vi "3_Axis_magmeter_MAIN.vi"() -> ()   [LabVIEW 2013]
doc: "Программа для обработки и визуализации трех компонент магнитного поля прибора, разработаного инженерами НЭОиКН ЛФВЭ ОИЯИ 2014"
uses:
  Magmeter.ctl
  <vilib>/Instr/_visa.llb/VISA Configure Serial Port (Instr).vi
panel:
  out "Dx Sum":u64
  in  "Порт":refnum<visa-resource-name>="COM4"
  out "Соединение":bool
  out "Err msg":string=" INSTRUCTIONS:\r\rNormal Use:  When using subVIs that incorporate the error in/error out (or error I/O) structure, place this handler where you want to inform the user of an error, typically at the end of the I/O data path, as the last action of the program.  If the error in error? is ERROR, the handler creates a message describing the error and its source.  If the type of dialog = 1 (default), the message is displayed to the user, who can only acknowedge it.  If the type = 2, the user can acknowledge the message or abort execution; aborting a program with active I/O is not recommended.  If the type = 0, no message is displayed; this is used to process the error programmatically, and the error out cluster elements are wired to individual terminals for that reason.  \r\rOther Use:\n\r\nlocal testing.  To test the error code of a subVI or function that does not have the error I/O structure, you can wire its error code and a source string to the local error code and error source inputs.  If error in error? indicates no error and error code is not equal to 0, the local code and source are substituted for the error in values, and error? is set TRUE (ERROR)."
  in  "Бод.":u32=9600
  out "i":i32
  in  "number of data sample":u64
  in  "Маркеры":bool
  out "Table num index":u32
  in  "Удалить измерение":bool
  in  "RXd number":u64
  in  "Dz, мм":u64=5 min=1
  in  "зафиксировать измерение":bool
  in  "Измерений \nна графике":u16=100
  in  "Очистить историю":bool
  in  "H макс":dbl=8.0 format="%#.1f"
  in  "H мин":dbl=-8.0 format="%#.1f"
  in  "Уст. ноль":bool
  in  "Сохранен!":bool
  in  "Plot.Visible Z":bool
  out "By":dbl format="%.3f"
  out "Bz":dbl format="%.3f"
  in  "Plot.Visible X":bool
  out "Bx":dbl format="%.3f"
  in  "Plot.Visible Y":bool
  in  "Графики толще":bool=TRUE
  in  "Scale Max, Ga":string(combo)="8,1"
  in  "Стоп":bool
  out "Магнитные измерения":T1(graph)
  in  "Measurment Fl":bool
  out "Сохраненные измерения":string[][](table)
  out "Путь к файлу":path
  # "Гаусс"
  # "Результаты\nизмерений"
  # "ГС"
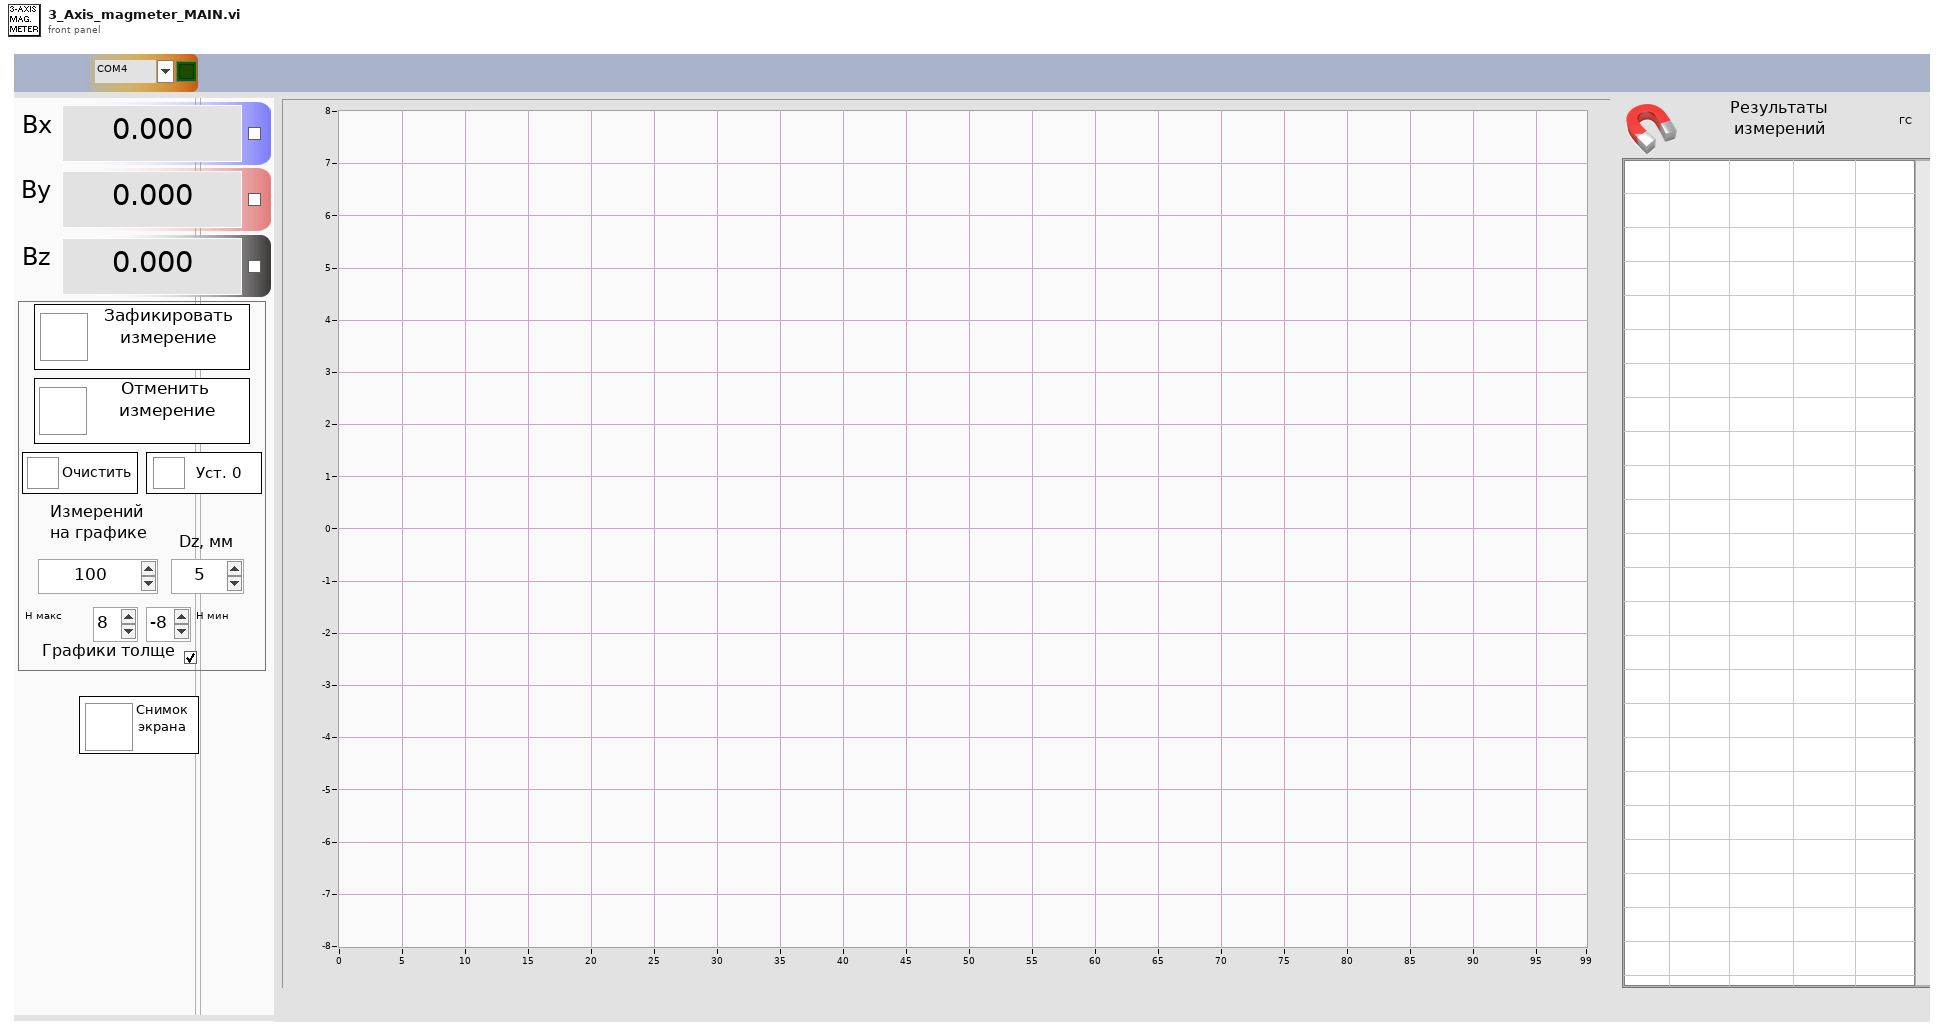
[diagram p1: front panel]
types:
  T1 = cluster{"X":dbl, "Y":dbl, "Z":dbl, "Active Plot":dbl}[]
  T2 = typedef "Magmeter.ctl" = enum16{"Initialize", "Read port", "Write port", "Stop"}
  T3 = cluster{"Value":dbl, "Value":dbl, "Value":dbl, "Active Plot":dbl}
  T4 = cluster{"Value":dbl, "Value":dbl, "Value":dbl, "X":dbl}
  T5 = cluster{"Value":dbl, "Value":dbl, "Value":dbl, "X":dbl}[]
  T6 = typedef "imagedata.ctl" = cluster{"image type":i32, "image depth":i32, "image":u8[], "mask":u8[], "colors":u32[], "Rectangle":cluster{"left":i16, "top":i16, "right":i16, "bottom":i16}}
  T7 = cluster{"read buffer":string, "serial out":refnum<visa-resource-name>, "error out":errorcluster, "occurrence":refnum<k4>}
  T8 = cluster{"Scale Max out ":string, "out string":string, "Visa name out":refnum<visa-resource-name>, "error out":errorcluster, "occurrence":refnum<k4>}
  T9 = cluster{"Visa name out":refnum<visa-resource-name>, "error out":errorcluster, "status":bool, "occurrence":refnum<k4>}
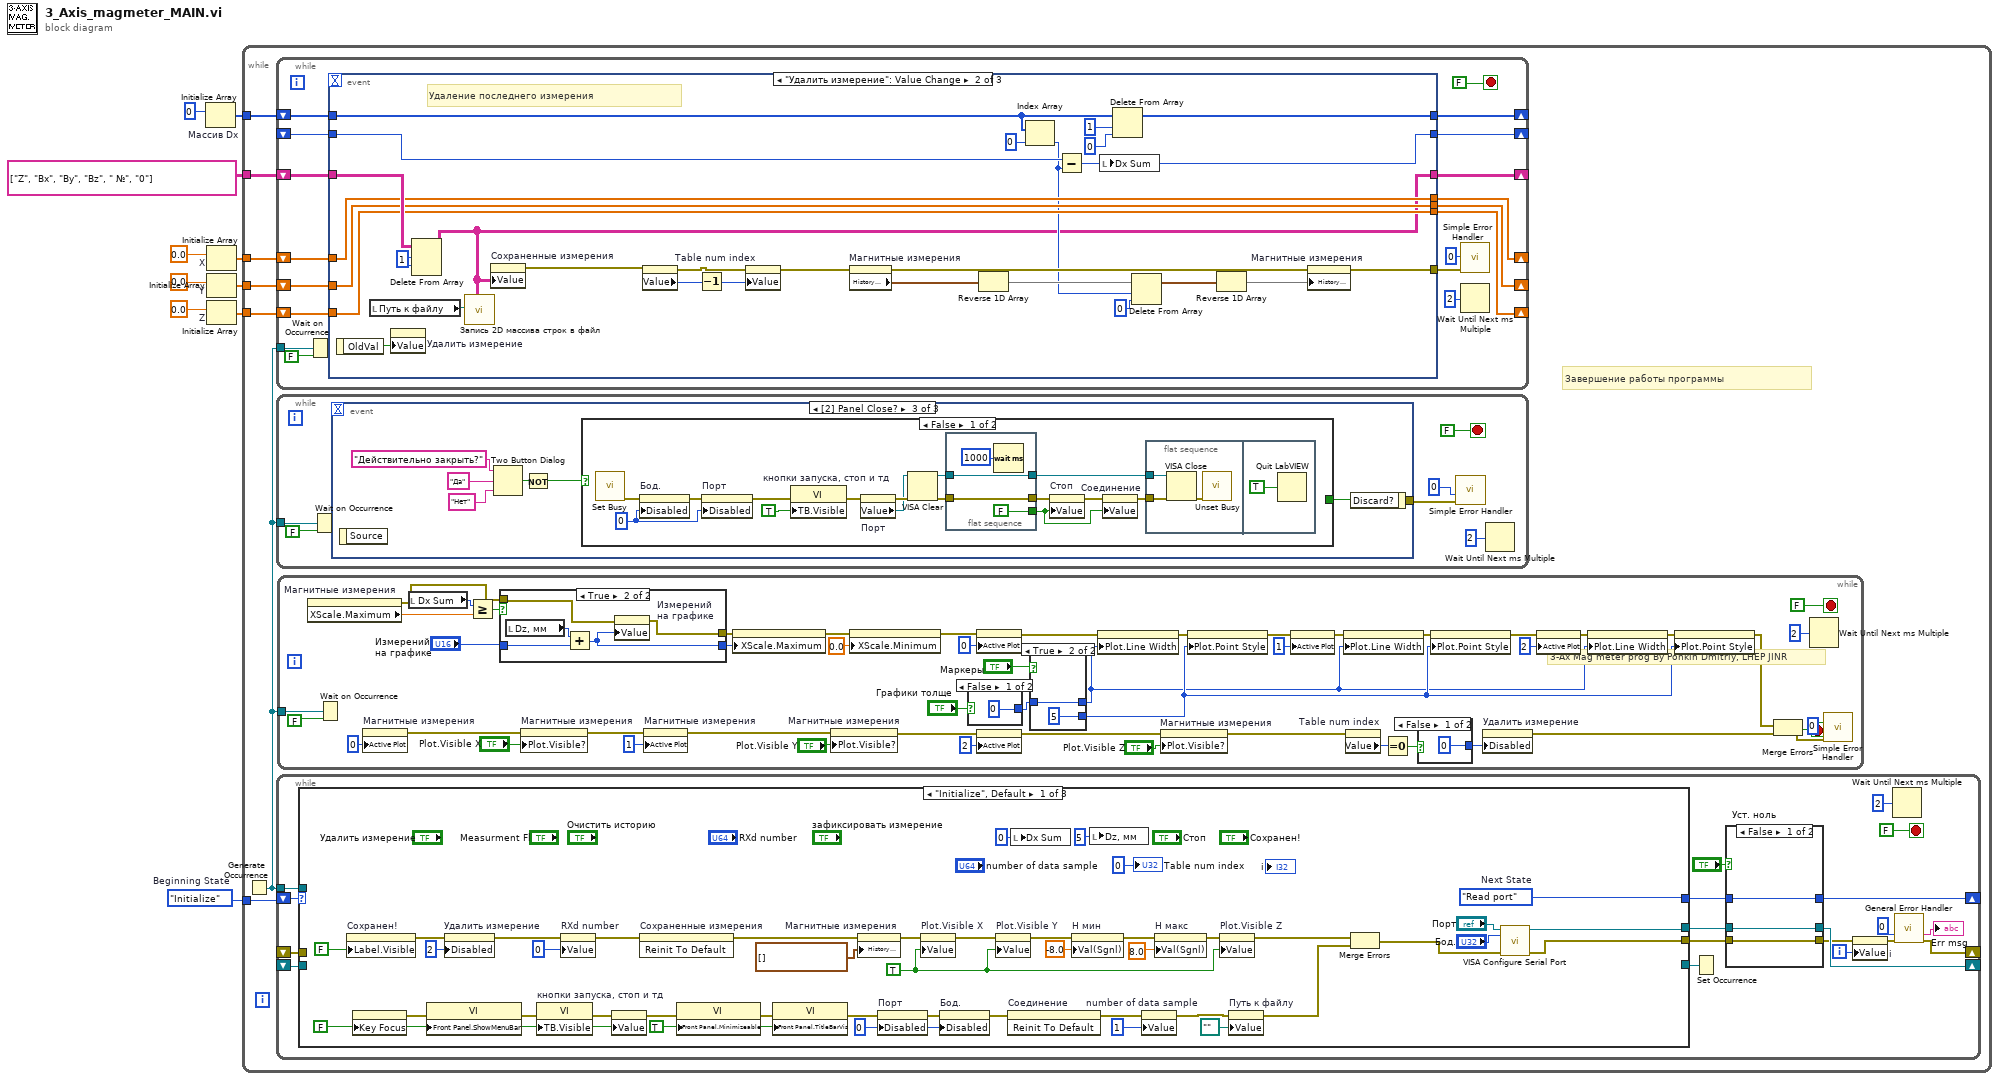
[diagram p0: block diagram]
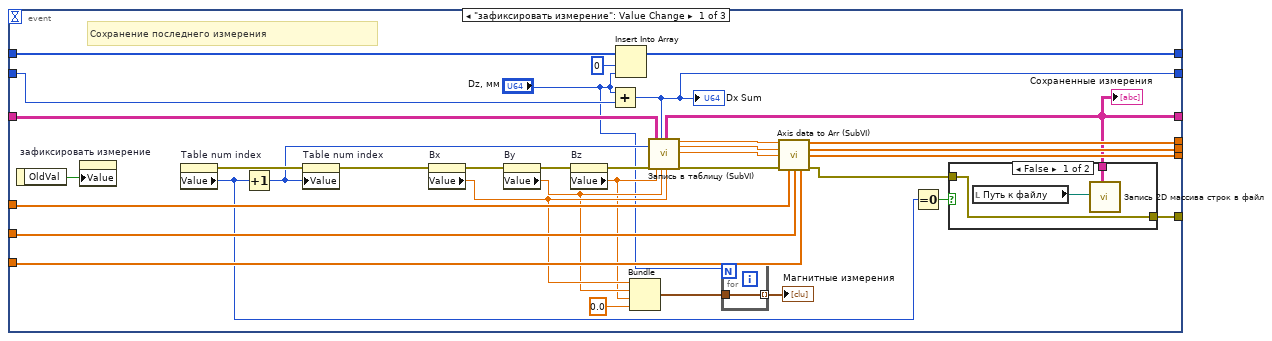
[diagram p2: hidden frame]
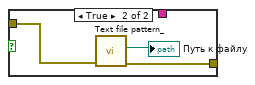
[diagram p3: hidden frame]
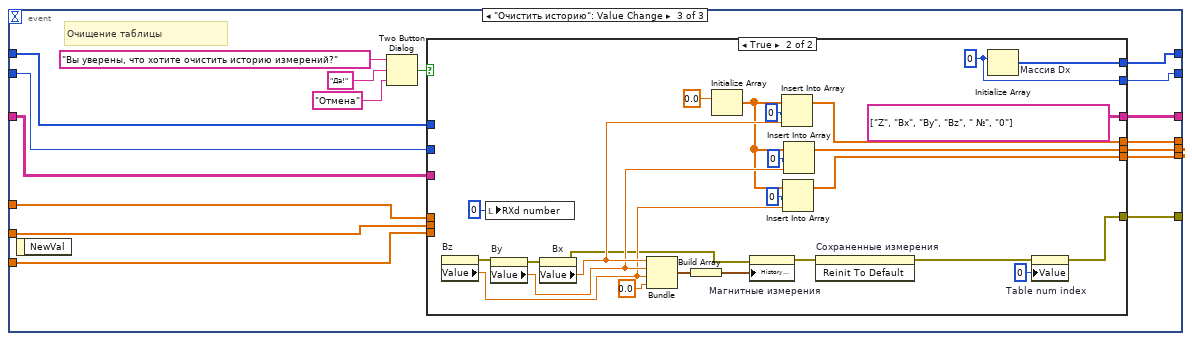
[diagram p4: hidden frame]
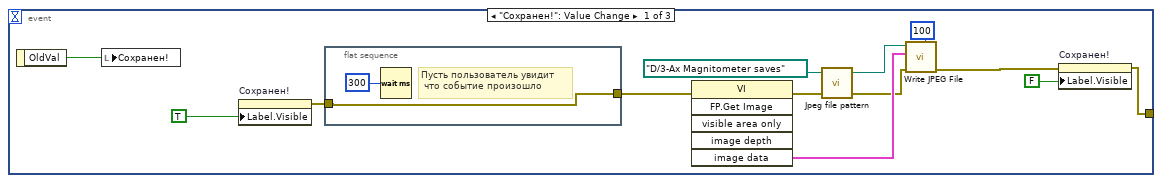
[diagram p6: hidden frame]
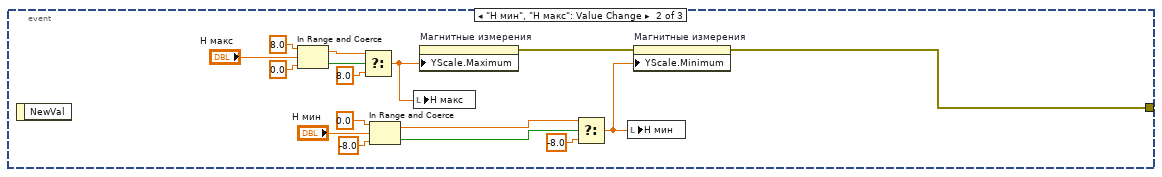
[diagram p7: hidden frame]
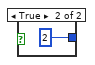
[diagram p9: hidden frame]
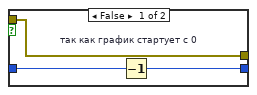
[diagram p10: hidden frame]
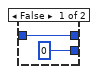
[diagram p11: hidden frame]
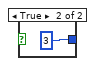
[diagram p12: hidden frame]
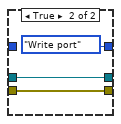
[diagram p13: hidden frame]
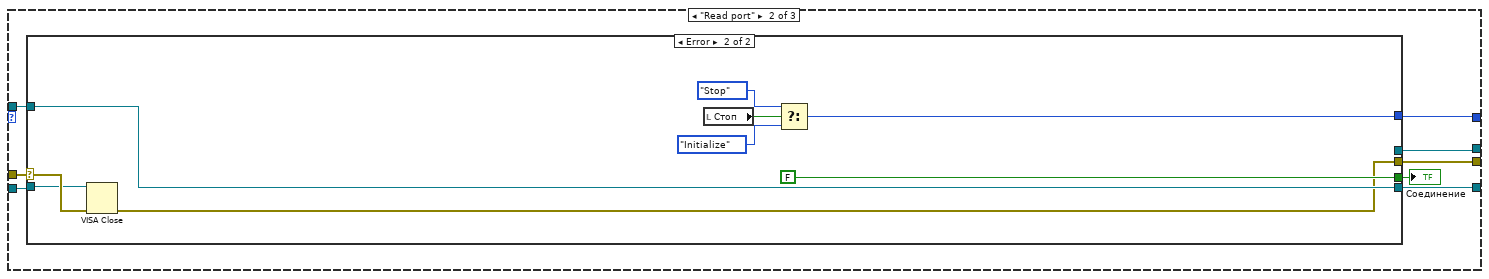
[diagram p14: hidden frame]
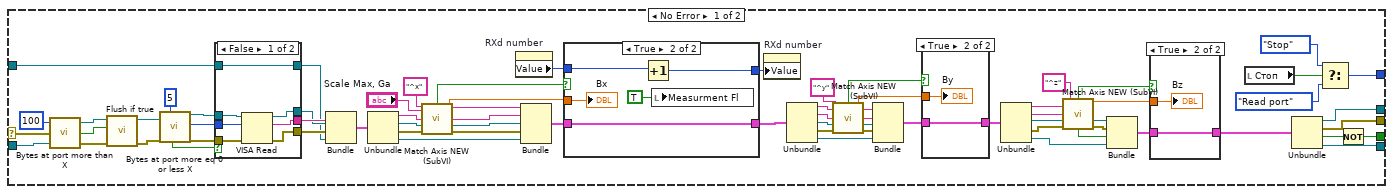
[diagram p15: hidden frame]
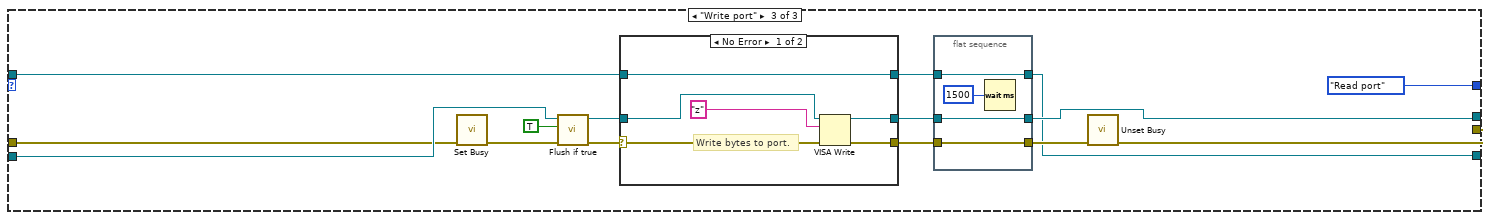
[diagram p20: hidden frame]
diagram:
  w10 = Magmeter."Initialize"  # Beginning State
  n1 = Initialize Array "Массив Dx"(u64 0 ("element")) -> (w1:u64[])  [unwired: 1 out]
  n2 = Initialize Array "X"(0.0 ("element")) -> (w7:dbl[])  [unwired: 1 out]
  n3 = Initialize Array "Y"(0.0 ("element")) -> (w4:dbl[])  [unwired: 1 out]
  n4 = Initialize Array "Z"(0.0 ("element")) -> (w3:dbl[])  [unwired: 1 out]
  n5 = while {
    tunnel: w10 -> [w18]
    tunnel: string[][] [["Z", "Bx", "By", "Bz", " №", "0"]] ("Сохраненные измерения") -> [w16]
    tunnel: w7 -> [w15]
    tunnel: w4 -> [w13]
    tunnel: w3 -> [w12]
    tunnel: w1 -> [w11]
    stop <- FALSE stop-if-true
    # "Завершение работы программы"
    # "3-Ax Mag meter prog By Ponkin Dmitriy, LHEP JINR"
    n6 = Generate Occurrence() -> (w14:refnum<k4>)
    n7 = while {
      shift-right: [w36] -> _
      shift-left: w16 -> [w35]
      shift-right: [w33] -> _
      shift-left: w15 -> [w34]
      tunnel: w14 -> [w30]
      shift-right: [w24] -> _
      shift-left: w12 -> [w26]
      shift-right: [w25] -> _
      shift-left: w13 -> [w27]
      shift-right: [w23] -> _
      shift-left: w11 -> [w22]
      shift-right: [w21] -> _
      shift-left: _ -> [w20]
      stop <- FALSE stop-if-true
      n8 = Wait on Occurrence(1:FALSE ("ignore previous (T)"), 2:w30) -> ()  [unwired: 1 in, 1 out]
      n9 = event shown="[1] \"Удалить измерение\": Value Change" {
        selector: _ -> [_ _ _]
        dyn-events: _ -> [_ _ _]
        timeout: _ -> [_ _ _]
        tunnel: w35 -> [w55 w104 w121]
        tunnel: [w37 w90 w122] -> w32
        tunnel: [w40 w80 w123] -> w36
        tunnel: w34 -> [w62 w102 w115]
        tunnel: [w59 w102 w116] -> w33
        tunnel: w27 -> [w61 w100 w114]
        tunnel: w26 -> [w60 w99 w113]
        tunnel: [w58 w99 w111] -> w24
        tunnel: [w57 w100 w112] -> w25
        tunnel: [w50 w87 w110] -> w23
        tunnel: w22 -> [w53 w82 w107]
        tunnel: [w52 w83 w109] -> w21
        tunnel: w20 -> [w51 w85 w108]
        event "зафиксировать измерение": Value Change {
          # "Сохранение последнего измерения"
          n10 = event-data() -> ("OldVal"=w47:bool)  [unwired: 1 out]
          n11 = property on="зафиксировать измерение" class="Bool (strict)"("Value"=w47) -> ()  [unwired: 2 in, 2 out]
          n12 = property on="Table num index" class="DigNum (strict)"() -> (error out=w71:errorcluster, "Value"=w39:u32)  [unwired: 2 in, 1 out]
          n13 = Increment(x=w39) -> (x+1=w56:u32)
          n14 = property on="Table num index" class="DigNum (strict)"(error in=w71, "Value"=w56) -> (error out=w68:errorcluster)  [unwired: 1 in, 1 out]
          n15 = property on="Bx" class="DigNum (strict)"(error in=w68) -> (error out=w70:errorcluster, "Value"=w46:dbl)  [unwired: 1 in, 1 out]
          n16 = property on="By" class="DigNum (strict)"(error in=w70) -> (error out=w69:errorcluster, "Value"=w45:dbl)  [unwired: 1 in, 1 out]
          n17 = property on="Bz" class="DigNum (strict)"(error in=w69) -> (error out=w67:errorcluster, "Value"=w44:dbl)  [unwired: 1 in, 1 out]
          n18 = Add(x="Dz, мм", y=w51) -> (x+y=w52:u64)
          "Dx Sum" <- w52
          n19 = Insert Into Array "Insert Into Array"(array=w53, index=0, new element="Dz, мм") -> (w50:u64[])
          n20 = Bundle("Value"=w46, "Value"=w45, "Value"=w44, "Active Plot"=0.0) -> (w49:T3)  [unwired: 1 out]
          n21 = call "Запись в таблицу (SubVI).vi"("data num"=w56, "error in"=w67, "String Arr in"=w55, "Z axis data"=w44, "Шаг измерений"=w52, "Y axis data"=w45, "X axis data"=w46) -> ("String Arr out"=w40:string[][], "X axis data out"=w65:dbl, "Y axis data out"=w64:dbl, "Z axis data out"=w63:dbl, "error out"=w66:errorcluster)  [unwired: 5 in, 3 out]
          "Сохраненные измерения" <- w40
          n22 = for {
            N: "Dz, мм" -> [_]
            tunnel: [w78] -> w42 mode=indexing
            tunnel: w49 -> [w78]
          }
          "Магнитные измерения" <- w42
          n23 = call "Axis data to Arr (SubVI).vi"("new X element"=w65, "new Y element"=w64, "new Z element"=w63, "error in"=w66, "X Arr in"=w62, "Y Arr in"=w61, "Z Arr in"=w60) -> ("X Arr Out"=w59:dbl[], "Y Arr Out"=w57:dbl[], "Z Arr Out"=w58:dbl[], "error out"=w38:errorcluster)  [unwired: 5 out]
          n24 = Equal To 0?(x=w39) -> (x = 0?=w41:bool)
          n25 = case shown="False" w41 {
            tunnel: w40 -> [w74 _]
            tunnel: w38 -> [w72 w76]
            tunnel: [w72 w75] -> w37
            frame False {
              n26 = local read "Путь к файлу"() -> (w73:path)
              n27 = call "Запись 2D массива строк в файл.vi"("путь к файлу"=w73, "2-D массив строк для записи"=w74) -> ()  [unwired: 2 in, 16 out]
            }
            frame True {
              n28 = call "Text file pattern_.vi"("error in"=w76) -> ("error out"=w75:errorcluster, "путь к файлу"=→"Путь к файлу":path)  [unwired: 9 out]
            }
          }
        }
        event "Удалить измерение": Value Change {
          w103 = 1 ("length")
          # "Удаление последнего измерения"
          n29 = event-data() -> ("OldVal"=w81:bool)  [unwired: 1 out]
          n30 = local read "Путь к файлу"() -> (w79:path)
          n31 = property on="Удалить измерение" class="Bool (strict)"("Value"=w81) -> ()  [unwired: 2 in, 2 out]
          n32 = Delete From Array "Delete From Array"(array=w104, length=w103, index (row)=w103) -> (array with subset deleted=w80:string[][])  [unwired: 1 in, 1 out]
          n33 = call "Запись 2D массива строк в файл.vi"("путь к файлу"=w79, "2-D массив строк для записи"=w80) -> ()  [unwired: 2 in, 16 out]
          n34 = property on="Сохраненные измерения" class="Tbl (strict)"("Value"=w80) -> (error out=w91:errorcluster)  [unwired: 2 in, 1 out]
          n35 = property on="Table num index" class="DigNum (strict)"(error in=w91) -> (error out=w101:errorcluster, "Value"=w106:u32)  [unwired: 1 in, 1 out]
          n36 = Decrement(x=w106) -> (x-1=w105:u32)
          n37 = property on="Table num index" class="DigNum (strict)"(error in=w101, "Value"=w105) -> (error out=w92:errorcluster)  [unwired: 1 in, 1 out]
          n38 = property on="Магнитные измерения" class="WFChart (strict)"(error in=w92) -> (error out=w93:errorcluster, "History Data"=w97:T1)  [unwired: 1 in, 1 out]
          n39 = Reverse 1D Array(array=w97) -> (reversed array=w96:T1)
          n40 = Index Array "Index Array"(array=w82, index=0) -> (element=w84:u64)
          n41 = Subtract(x=w85, y=w84) -> (x-y=w83:u64)
          n42 = local write "Dx Sum"(w83) -> ()
          n43 = Delete From Array "Delete From Array"(array=w82, length=1, index=0 ("length")) -> (array with subset deleted=w87:u64[])  [unwired: 1 out]
          n44 = Delete From Array "Delete From Array"(array=w96, length=w84, index=0 ("length")) -> (array with subset deleted=w94:T1)  [unwired: 1 out]
          n45 = Reverse 1D Array(array=w94) -> (reversed array=w95:T1)
          n46 = property on="Магнитные измерения" class="WFChart (strict)"(error in=w93, "History Data"=w95) -> (error out=w90:errorcluster)  [unwired: 1 in, 1 out]
        }
        event "Очистить историю": Value Change {
          # "Очищение таблицы"
          n47 = event-data() -> ()  [unwired: 2 out]
          n48 = Two Button Dialog(message="Вы уверены, что хотите очистить историю измерений?", 1:"Отмена" ("T button name (\"OK\")"), 2:"Да!" ("T button name (\"OK\")")) -> (T button?=w117:bool)
          n49 = case shown="True" w117 {
            tunnel: [w129 string[][] [["Z", "Bx", "By", "Bz", " №", "0"]] ("Сохраненные измерения")] -> w123
            tunnel: [_ w133] -> w122
            tunnel: w121 -> [w129 _]
            tunnel: [w128 w146] -> w116
            tunnel: w115 -> [w128 _]
            tunnel: w114 -> [w127 _]
            tunnel: w113 -> [w126 _]
            tunnel: [w127 w141] -> w112
            tunnel: [w126 w139] -> w111
            tunnel: w107 -> [w125 _]
            tunnel: [w125 w132] -> w110
            tunnel: [w124 w131] -> w109
            tunnel: w108 -> [w124 _]
            frame False {
            }
            frame True {
              w131 = u64 0 ("element")
              n50 = property on="Bz" class="DigNum (strict)"() -> (error out=w136:errorcluster, "Value"=w138:dbl)  [unwired: 2 in, 1 out]
              n51 = local write "RXd number"(u64 0 ("RXd number")) -> ()
              n52 = property on="By" class="DigNum (strict)"(error in=w136) -> (error out=w135:errorcluster, "Value"=w142:dbl)  [unwired: 1 in, 1 out]
              n53 = property on="Bx" class="DigNum (strict)"(error in=w135) -> (error out=w134:errorcluster, "Value"=w143:dbl)  [unwired: 1 in, 1 out]
              n54 = Bundle("Value"=w143, "Value"=w142, "Value"=w138, "X"=0.0) -> (w149:T4)  [unwired: 1 out]
              n55 = Build Array(w149) -> (w144:T5)
              n56 = Initialize Array(0.0 ("element")) -> (w137:dbl[])  [unwired: 1 out]
              n57 = property on="Магнитные измерения" class="WFChart (strict)"(error in=w134, "History Data"=w144) -> (error out=w151:errorcluster)  [unwired: 1 in, 1 out]
              n58 = Insert Into Array(array=w137, index=0, new element=w143) -> (w146:dbl[])
              n59 = Insert Into Array(array=w137, index=0, new element=w138) -> (w139:dbl[])
              n60 = Insert Into Array(array=w137, index=0, new element=w142) -> (w141:dbl[])
              n61 = invoke on="Сохраненные измерения" class="Tbl (strict)" method="Reinit To Default"(error in=w151) -> (error out=w153:errorcluster)  [unwired: 2 in, 2 out]
              n62 = Initialize Array "Массив Dx"(w131) -> (w132:u64[])  [unwired: 1 out]
              n63 = property on="Table num index" class="DigNum (strict)"(error in=w153, "Value"=u32 0 ("Table num index")) -> (error out=w133:errorcluster)  [unwired: 1 in, 1 out]
            }
          }
        }
      }
      n64 = call <vilib>:"Simple Error Handler.vi"("type of dialog (OK msg:1)"=u32 0 ("Table num index"), "error in (no error)"=w32) -> ()  [unwired: 8 out]
      n65 = Wait Until Next ms Multiple(millisecond multiple=u32 2) -> ()  [unwired: 1 out]
    }
    n66 = while {
      tunnel: w14 -> [w157]
      stop <- FALSE stop-if-true
      n67 = Wait on Occurrence(1:FALSE ("ignore previous (T)"), 2:w157) -> ()  [unwired: 1 in, 1 out]
      n68 = event shown="[2] Panel Close?" {
        selector: _ -> [_ _ _]
        dyn-events: _ -> [_ _ _]
        timeout: _ -> [_ _ _]
        tunnel: [w167 w176 _] -> w159
        event "Сохранен!": Value Change {
          n69 = event-data() -> ("OldVal"=w168:bool)  [unwired: 1 out]
          n70 = local write "Сохранен!"(w168) -> ()
          n71 = property on="Сохранен!" class="Bool (strict)"("Label.Visible"=TRUE) -> (error out=w162:errorcluster)  [unwired: 2 in, 1 out]
          n72 = flat-sequence {
            tunnel: [w174] -> w163
            tunnel: w162 -> [w174]
            frame #0 {
              # "Пусть пользователь увидит\n что событие произошло"
              n73 = Wait (ms)(milliseconds to wait=u32 300) -> ()  [unwired: 1 out]
            }
          }
          n74 = invoke class="VI" method="FP.Get Image"(error in=w163) -> (error out=w171:errorcluster, "image data"=w172:T6)  [unwired: 5 in, 4 out]
          n75 = call "Jpeg file pattern.vi"("path"=path "D:/3-Ax Magnitometer saves" ("path (use dialog)"), "error in"=w171) -> ("path to JPG file"=w170:path, "error out"=w169:errorcluster)  [unwired: 6 out]
          n76 = call <vilib>:"Write JPEG File.vi"("quality (80)"=100, "error in (no error)"=w169, "image data"=w172, "path to JPEG file"=w170) -> ("error out"=w166:errorcluster)  [unwired: 7 out]
          n77 = property on="Сохранен!" class="Bool (strict)"(error in=w166, "Label.Visible"=FALSE) -> (error out=w167:errorcluster)  [unwired: 1 in, 1 out]
        }
        event "H мин", "H макс": Value Change {
          n78 = event-data() -> ()  [unwired: 2 out]
          n79 = In Range and Coerce(upper limit=8.0, x="H макс", lower limit=0.0) -> (coerced(x)=w187:dbl, In Range?=w189:bool)
          n80 = Select(t=w187, s=w189, f=8.0) -> (s? t:f=w179:dbl)
          n81 = In Range and Coerce(upper limit=0.0, x="H мин", lower limit=-8.0) -> (coerced(x)=w185:dbl, In Range?=w183:bool)
          n82 = local write "H макс"(w179) -> ()
          n83 = property on="Магнитные измерения" class="WFChart (strict)"("YScale.Maximum"=w179) -> (error out=w177:errorcluster)  [unwired: 2 in, 1 out]
          n84 = Select(t=w185, s=w183, f=-8.0) -> (s? t:f=w178:dbl)
          n85 = local write "H мин"(w178) -> ()
          n86 = property on="Магнитные измерения" class="WFChart (strict)"(error in=w177, "YScale.Minimum"=w178) -> (error out=w176:errorcluster)  [unwired: 1 in, 1 out]
        }
        event Panel Close? {
          n87 = event-data() -> ()  [unwired: 2 out]
          n88 = Two Button Dialog(message="Действительно закрыть?", 1:"Нет", 2:"Да") -> (T button?=w194:bool)
          n89 = Not(x=w194) -> (.not. x?=w193:bool)
          n90 = case shown="False" w193 {
            selector: w193 -> [_ w221]
            tunnel: [_ w221] -> w192
            frame False {
              w208 = u8 0 ("Disabled")
              n91 = call <vilib>:"Set Busy.vi"() -> ("error out"=w198:errorcluster)  [unwired: 4 in, 7 out]
              n92 = property on="Бод." class="DigNum (strict)"(error in=w198, "Disabled"=w208) -> (error out=w211:errorcluster)  [unwired: 1 in, 1 out]
              n93 = property on="Порт" class="VISAName"(error in=w211, "Disabled"=w208) -> (error out=w202:errorcluster)  [unwired: 1 in, 1 out]
              n94 = property on="кнопки запуска, стоп и тд" class="VI"(error in=w202, "TB.Visible"=TRUE ("Tool Bar:Visible")) -> (error out=w200:errorcluster)  [unwired: 1 in, 1 out]
              n95 = property on="Порт" class="VISAName"(error in=w200) -> (error out=w201:errorcluster, "Value"=w199:refnum<visa-resource-name>)  [unwired: 1 in, 1 out]
              n96 = VISA Clear(VISA resource name=w199, error in (no error)=w201) -> (VISA resource name out=w210:refnum<visa-resource-name>, error out=w209:errorcluster)
              n97 = flat-sequence {
                tunnel: w210 -> [w215]
                tunnel: [w215] -> w206
                tunnel: [w214] -> w204
                tunnel: w209 -> [w214]
                tunnel: [FALSE ("Visible")] -> w203
                frame #0 {
                  n98 = Wait (ms)(milliseconds to wait=u32 1000) -> ()  [unwired: 1 out]
                }
              }
              n99 = property on="Стоп" class="Bool (strict)"(error in=w204, "Value"=w203) -> (error out=w205:errorcluster)  [unwired: 1 in, 1 out]
              n100 = property on="Соединение" class="Bool (strict)"(error in=w205, "Value"=w203) -> (error out=w207:errorcluster)  [unwired: 1 in, 1 out]
              n101 = flat-sequence {
                tunnel: w207 -> [w219]
                tunnel: w206 -> [w218]
                frame #0 {
                  n102 = VISA Close(VISA resource name=w218, error in (no error)=w219) -> (error out=w217:errorcluster)
                  n103 = call <vilib>:"Unset Busy.vi"("error in (no error)"=w217) -> ()  [unwired: 1 in, 10 out]
                }
                frame #1 {
                  n104 = Quit LabVIEW(quit? (T)=TRUE ("stop? (T)")) -> ()
                }
              }
            }
            frame True {
            }
          }
          n105 = event-data("Discard?"=w192) -> ()  [unwired: 1 in, 1 out]
        }
      }
      n106 = call <vilib>:"Simple Error Handler.vi"("type of dialog (OK msg:1)"=u32 0 ("Table num index"), "error in (no error)"=w159) -> ()  [unwired: 8 out]
      n107 = Wait Until Next ms Multiple(millisecond multiple=u32 2) -> ()  [unwired: 1 out]
    }
    n108 = while "While sa" {
      shift-right: [w296] -> _
      shift-left: w18 -> [w305]
      shift-right: [w288] -> _
      shift-left: _ -> [w302]
      tunnel: w14 -> [w299]
      shift-right: [w294] -> _
      shift-left: _ -> [w298]
      i -> [w301]
      stop <- FALSE stop-if-true
      n109 = case shown="\"Initialize\", Default" w305 {
        tunnel: [w348 w355 Magmeter."Read port" ("Beginning State")] -> w297
        tunnel: w302 -> [_ w358 w472]
        tunnel: w299 -> [_ w360 w476]
        tunnel: w298 -> [_ w359 w474]
        tunnel: [w332 w354 w466] -> w293
        tunnel: [w331 w357 w471] -> w291
        tunnel: [_ w356 w465] -> w292
        frame "Initialize", Default {
          w348 = Magmeter."Read port"  # Next State
          w335 = TRUE ("Plot.Visible X")
          w345 = TRUE ("Front Panel Window:Minimizable")
          w342 = FALSE ("Front Panel Window:Resizable")
          w343 = u8 0 ("Disabled")
          n110 = property on="Сохранен!" class="Bool (strict)"("Label.Visible"=FALSE) -> (error out=w325:errorcluster)  [unwired: 2 in, 1 out]
          n111 = property on="Стоп" class="Bool (strict)"("Key Focus"=w342) -> (error out=w347:errorcluster)  [unwired: 2 in, 1 out]
          n112 = property class="VI"(error in=w347, "Front Panel.ShowMenuBar"=w342) -> (error out=w346:errorcluster)  [unwired: 1 in, 1 out]
          n113 = property on="Удалить измерение" class="Bool (strict)"(error in=w325, "Disabled"=u8 2) -> (error out=w327:errorcluster)  [unwired: 1 in, 1 out]
          n114 = property on="кнопки запуска, стоп и тд" class="VI"(error in=w346, "TB.Visible"=w342) -> (error out=w341:errorcluster)  [unwired: 1 in, 1 out]
          n115 = property on="RXd number" class="DigNum (strict)"(error in=w327, "Value"=u64 0 ("RXd number")) -> (error out=w328:errorcluster)  [unwired: 1 in, 1 out]
          n116 = property on="Стоп" class="Bool (strict)"(error in=w341, "Value"=w342) -> (error out=w338:errorcluster)  [unwired: 1 in, 1 out]
          n117 = invoke on="Сохраненные измерения" class="Tbl (strict)" method="Reinit To Default"(error in=w328) -> (error out=w329:errorcluster)  [unwired: 2 in, 2 out]
          n118 = property class="VI"(error in=w338, "Front Panel.Minimizeable"=w345) -> (error out=w344:errorcluster)  [unwired: 1 in, 1 out]
          n119 = property class="VI"(error in=w344, "Front Panel.TitleBarVis"=w345) -> (error out=w339:errorcluster)  [unwired: 1 in, 1 out]
          n120 = property on="Магнитные измерения" class="WFChart (strict)"(error in=w329, "History Data"=T1 []) -> (error out=w333:errorcluster)  [unwired: 1 in, 1 out]
          n121 = property on="Порт" class="VISAName"(error in=w339, "Disabled"=w343) -> (error out=w340:errorcluster)  [unwired: 1 in, 1 out]
          n122 = property on="Plot.Visible X" class="Bool (strict)"(error in=w333, "Value"=w335) -> (error out=w336:errorcluster)  [unwired: 1 in, 1 out]
          n123 = property on="Бод." class="DigNum (strict)"(error in=w340, "Disabled"=w343) -> (error out=w349:errorcluster)  [unwired: 1 in, 1 out]
          n124 = property on="Plot.Visible Y" class="Bool (strict)"(error in=w336, "Value"=w335) -> (error out=w322:errorcluster)  [unwired: 1 in, 1 out]
          n125 = invoke on="Соединение" class="Bool (strict)" method="Reinit To Default"(error in=w349) -> (error out=w352:errorcluster)  [unwired: 2 in, 2 out]
          n126 = local write "Dx Sum"(u64 0 ("Dx Sum")) -> ()
          n127 = property on="H мин" class="DigNum (strict)"(error in=w322, "Val(Sgnl)"=-8.0 ("Value (Signaling)")) -> (error out=w320:errorcluster)  [unwired: 1 in, 1 out]
          n128 = local write "Dz, мм"(u64 5 ("Dz, мм")) -> ()
          n129 = property on="number of data sample" class="DigNum (strict)"(error in=w352, "Value"=u64 1 ("number of data sample")) -> (error out=w313:errorcluster)  [unwired: 1 in, 1 out]
          n130 = property on="H макс" class="DigNum (strict)"(error in=w320, "Val(Sgnl)"=8.0 ("Value (Signaling)")) -> (error out=w319:errorcluster)  [unwired: 1 in, 1 out]
          n131 = property on="Plot.Visible Z" class="Bool (strict)"(error in=w319, "Value"=w335) -> (error out=w316:errorcluster)  [unwired: 1 in, 1 out]
          n132 = property on="Путь к файлу" class="Path"(error in=w313, "Value"=path "" ("Путь к файлу")) -> (error out=w312:errorcluster)  [unwired: 1 in, 1 out]
          n133 = Merge Errors(w316, w312) -> (w315:errorcluster)
          n134 = call-poly "VISA Configure Serial Port"("VISA resource name"="Порт", "baud rate (9600)"="Бод.", "error in (no error)"=w315) -> ("VISA resource name out"=w332:refnum<visa-resource-name>, "error out"=w331:errorcluster)  [unwired: 3 in, 8 out]
          "Table num index" <- u32 0 ("Table num index")
        }
        frame "Read port" {
          n135 = case shown="Error" w358 {
            selector: w358 -> [w409 w463]
            tunnel: [w430 w459] -> w355
            tunnel: [w367 FALSE] -> w361
            tunnel: w360 -> [w362 w458]
            tunnel: w359 -> [w368 w457]
            tunnel: [w371 _] -> w354
            tunnel: [w364 w456] -> w357
            tunnel: [w369 w458] -> w356
            frame No Error {
              n136 = call "Bytes at port more than X.vi"("X"=u32 100, "error IO"=w409, "port in"=w368) -> ("port out"=w408:refnum<visa-resource-name>, "Bytes at port > X"=w429:bool, "error out"=w407:errorcluster)  [unwired: 1 in, 3 out]
              n137 = call "Flush if true.vi"("error in"=w407, "Bytes at port > X"=w429, "port in"=w408) -> ("error out"=w428:errorcluster, "port out"=w427:refnum<visa-resource-name>)  [unwired: 1 in, 6 out]
              n138 = call "Bytes at port more eq 0 or less X.vi"("X"=u32 5, "serial ref  name"=w427, "error IO"=w428) -> ("Bytes at port <X or = 0?"=w375:bool, "serial out"=w423:refnum<visa-resource-name>, "Num. of Bytes at Port"=w425:u32, "error out"=w424:errorcluster)  [unwired: 2 in, 11 out]
              n139 = case shown="False" w375 {
                tunnel: w424 -> [w452 w454]
                tunnel: w425 -> [w451 _]
                tunnel: w423 -> [w450 w455]
                tunnel: [w449 w455] -> w420
                tunnel: [w448 _] -> w421
                tunnel: [w447 w454] -> w366
                tunnel: [w446 w453] -> w363
                tunnel: w362 -> [w446 w453]
                frame False {
                  n140 = VISA Read(VISA resource name=w450, byte count=w451, error in (no error)=w452) -> (VISA resource name out=w449:refnum<visa-resource-name>, read buffer=w448:string, error out=w447:errorcluster)  [unwired: 1 out]
                }
                frame True {
                }
              }
              n141 = Bundle("read buffer"=w421, "serial out"=w420, "error out"=w366, "occurrence"=w363) -> (w365:T7)  [unwired: 1 out]
              n142 = Unbundle(w365) -> ("read buffer"=w415:string, "serial out"=w414:refnum<visa-resource-name>, "error out"=w422:errorcluster, "occurrence"=w382:refnum<k4>)
              n143 = call "Match Axis NEW (SubVI).vi"("Axis ID"="^x", "Scale Max, Ga"="Scale Max, Ga", "input string"=w415, "Visa name in"=w414, "error in"=w422) -> ("Good\nto read!"=w405:bool, "out number"=w417:dbl, "Scale Max out"=w402:string, "out string"=w401:string, "Visa name out"=w400:refnum<visa-resource-name>, "error out"=w399:errorcluster)  [unwired: 1 in, 4 out]
              n144 = property on="RXd number" class="DigNum (strict)"() -> ("Value"=w373:u64)  [unwired: 2 in, 2 out]
              n145 = Bundle("Scale Max out"=w402, "out string"=w401, "Visa name out"=w400, "error out"=w399, "occurrence"=w382) -> (w398:T8)  [unwired: 1 out]
              n146 = case shown="True" w405 {
                tunnel: w417 -> [_ w442]
                tunnel: w398 -> [w440 w445]
                tunnel: [w440 w445] -> w397
                tunnel: [w439 w443] -> w374
                tunnel: w373 -> [w439 w444]
                frame False {
                }
                frame True {
                  n147 = Increment(x=w444) -> (x+1=w443:u64)
                  n148 = local write "Measurment Fl"(TRUE ("Measurment Fl")) -> ()
                  "Bx" <- w442
                }
              }
              n149 = property on="RXd number" class="DigNum (strict)"("Value"=w374) -> ()  [unwired: 2 in, 2 out]
              n150 = Unbundle(w397) -> ("Scale Max out"=w396:string, "out string"=w395:string, "Visa name out"=w394:refnum<visa-resource-name>, "error out"=w393:errorcluster, "occurrence"=w381:refnum<k4>)
              n151 = call "Match Axis NEW (SubVI).vi"("Axis ID"="^y", "Scale Max, Ga"=w396, "input string"=w395, "Visa name in"=w394, "error in"=w393) -> ("Good\nto read!"=w404:bool, "out number"=w413:dbl, "Scale Max out"=w392:string, "out string"=w391:string, "Visa name out"=w390:refnum<visa-resource-name>, "error out"=w389:errorcluster)  [unwired: 1 in, 4 out]
              n152 = Bundle("Scale Max out"=w392, "out string"=w391, "Visa name out"=w390, "error out"=w389, "occurrence"=w381) -> (w388:T8)  [unwired: 1 out]
              n153 = case shown="True" w404 {
                tunnel: w413 -> [_ w437]
                tunnel: w388 -> [w436 w438]
                tunnel: [w436 w438] -> w387
                frame False {
                }
                frame True {
                  "By" <- w437
                }
              }
              n154 = Unbundle(w387) -> ("Scale Max out"=w386:string, "out string"=w385:string, "Visa name out"=w384:refnum<visa-resource-name>, "error out"=w383:errorcluster, "occurrence"=w377:refnum<k4>)
              n155 = call "Match Axis NEW (SubVI).vi"("Axis ID"="^z", "Scale Max, Ga"=w386, "input string"=w385, "Visa name in"=w384, "error in"=w383) -> ("Good\nto read!"=w403:bool, "out number"=w411:dbl, "Visa name out"=w380:refnum<visa-resource-name>, "status"=w378:bool, "error out"=w379:errorcluster)  [unwired: 1 in, 5 out]
              n156 = Bundle("Visa name out"=w380, "error out"=w379, "status"=w378, "occurrence"=w377) -> (w376:T9)  [unwired: 1 out]
              n157 = case shown="True" w403 {
                tunnel: w411 -> [_ w434]
                tunnel: w376 -> [w433 w435]
                tunnel: [w433 w435] -> w372
                frame False {
                }
                frame True {
                  "Bz" <- w434
                }
              }
              n158 = local read "Стоп"() -> (w426:bool)
              n159 = Unbundle(w372) -> ("Visa name out"=w371:refnum<visa-resource-name>, "error out"=w364:errorcluster, "status"=w370:bool, "occurrence"=w369:refnum<k4>)
              n160 = Select(t=Magmeter."Stop" ("Beginning State"), s=w426, f=Magmeter."Read port" ("Beginning State")) -> (s? t:f=w430:T2)
              n161 = Not(x=w370) -> (.not. x?=w367:bool)
            }
            frame Error {
              n162 = VISA Close(VISA resource name=w457, error in (no error)=w463) -> (error out=w456:errorcluster)
              n163 = local read "Стоп"() -> (w462:bool)
              n164 = Select(t=Magmeter."Stop" ("Beginning State"), s=w462, f=Magmeter."Initialize" ("Beginning State")) -> (s? t:f=w459:T2)
            }
          }
          "Соединение" <- w361
        }
        frame "Write port" {
          n165 = call <vilib>:"Set Busy.vi"("error in (no error)"=w472) -> ("error out"=w473:errorcluster)  [unwired: 3 in, 7 out]
          n166 = call "Flush if true.vi"("error in"=w473, "Bytes at port > X"=TRUE, "port in"=w474) -> ("error out"=w479:errorcluster, "port out"=w478:refnum<visa-resource-name>)  [unwired: 1 in, 6 out]
          n167 = case shown="No Error" w479 {
            selector: w479 -> [w487 w492]
            tunnel: [w489 w491] -> w470
            tunnel: [w488 w492] -> w469
            tunnel: w478 -> [w486 w491]
            tunnel: w476 -> [w484 w490]
            tunnel: [w484 w490] -> w467
            frame No Error {
              # "Write bytes to port."
              n168 = VISA Write(VISA resource name=w486, write buffer="z", error in (no error)=w487) -> (VISA resource name out=w489:refnum<visa-resource-name>, error out=w488:errorcluster)  [unwired: 1 out]
            }
            frame Error {
            }
          }
          n169 = flat-sequence {
            tunnel: w470 -> [w483]
            tunnel: [w483] -> w466
            tunnel: w469 -> [w482]
            tunnel: [w482] -> w468
            tunnel: w467 -> [w481]
            tunnel: [w481] -> w465
            frame #0 {
              n170 = Wait (ms)(milliseconds to wait=u32 1500) -> ()  [unwired: 1 out]
            }
          }
          n171 = call <vilib>:"Unset Busy.vi"("error in (no error)"=w468) -> ("error out"=w471:errorcluster)  [unwired: 1 in, 9 out]
        }
      }
      n172 = Set Occurrence(w292) -> ()
      n173 = case shown="False" "Уст. ноль" {
        tunnel: w297 -> [w308 _]
        tunnel: [w308 Magmeter."Write port" ("Beginning State")] -> w296
        tunnel: [w307 w310] -> w294
        tunnel: w293 -> [w307 w310]
        tunnel: w291 -> [w306 w309]
        tunnel: [w306 w309] -> w290
        frame False {
        }
        frame True {
        }
      }
      n174 = property on="i" class="DigNum (strict)"(error in=w290, "Value"=w301) -> (error out=w300:errorcluster)  [unwired: 1 in, 1 out]
      n175 = Wait Until Next ms Multiple(millisecond multiple=u32 2) -> ()  [unwired: 1 out]
      n176 = call <vilib>:"General Error Handler.vi"("type of dialog (OK msg:1)"=u8 0 ("Disabled"), "error in (no error)"=w300) -> ("message"=→"Err msg":string, "error out"=w288:errorcluster)  [unwired: 12 out]
    }
    n177 = while {
      tunnel: w14 -> [w261]
      stop <- FALSE stop-if-true
      n178 = property on="Магнитные измерения" class="WFChart (strict)"() -> (error out=w229:errorcluster, "XScale.Maximum"=w235:dbl)  [unwired: 2 in, 1 out]
      n179 = Wait on Occurrence(1:FALSE ("ignore previous (T)"), 2:w261) -> ()  [unwired: 1 in, 1 out]
      n180 = property on="Магнитные измерения" class="WFChart (strict)"("Active Plot"=u32 0) -> (error out=w240:errorcluster)  [unwired: 2 in, 1 out]
      n181 = local read "Dx Sum"() -> (w237:u64)
      n182 = Greater Or Equal?(x=w237, y=w235) -> (x >= y?=w236:bool)
      n183 = case shown="True" w236 {
        tunnel: [w275 w279] -> w238
        tunnel: "Измерений \nна графике" -> [w274 w278]
        tunnel: w229 -> [w273 w277]
        tunnel: [w273 w276] -> w228
        frame False {
          n184 = Decrement "так как график стартует с 0"(x=w274) -> (x-1=w275:u16)
        }
        frame True {
          n185 = local read "Dz, мм"() -> (w280:u64)
          n186 = Add(x=w280, y=w278) -> (x+y=w279:u64)
          n187 = property on="Измерений \nна графике" class="DigNum (strict)"(error in=w277, "Value"=w279) -> (error out=w276:errorcluster)  [unwired: 1 in, 1 out]
        }
      }
      n188 = property on="Магнитные измерения" class="WFChart (strict)"(error in=w240, "Plot.Visible?"="Plot.Visible X") -> (error out=w263:errorcluster)  [unwired: 1 in, 1 out]
      n189 = property on="Магнитные измерения" class="WFChart (strict)"(error in=w263, "Active Plot"=u32 1) -> (error out=w259:errorcluster)  [unwired: 1 in, 1 out]
      n190 = property on="Магнитные измерения" class="WFChart (strict)"(error in=w228, "XScale.Maximum"=w238) -> (error out=w241:errorcluster)  [unwired: 1 in, 1 out]
      n191 = property on="Магнитные измерения" class="WFChart (strict)"(error in=w259, "Plot.Visible?"="Plot.Visible Y") -> (error out=w243:errorcluster)  [unwired: 1 in, 1 out]
      n192 = property on="Магнитные измерения" class="WFChart (strict)"(error in=w241, "XScale.Minimum"=0.0 ("X Scale.Range:Minimum")) -> (error out=w239:errorcluster)  [unwired: 1 in, 1 out]
      n193 = case shown="False" "Графики толще" {
        tunnel: [u8 0 ("Plot.Line Width") u8 3 ("Plot.Line Width")] -> w247
        frame False {
        }
        frame True {
        }
      }
      n194 = property on="Магнитные измерения" class="WFChart (strict)"(error in=w239, "Active Plot"=u32 0) -> (error out=w242:errorcluster)  [unwired: 1 in, 1 out]
      n195 = property on="Магнитные измерения" class="WFChart (strict)"(error in=w243, "Active Plot"=u32 2) -> (error out=w265:errorcluster)  [unwired: 1 in, 1 out]
      n196 = case shown="True" "Маркеры" {
        tunnel: [w282 w284] -> w233
        tunnel: w247 -> [w282 w284]
        tunnel: [u8 0 ("Plot.Line Width") u8 5 ("Plot.Line Width")] -> w245
        frame False {
        }
        frame True {
        }
      }
      n197 = property on="Магнитные измерения" class="WFChart (strict)"(error in=w242, "Plot.Line Width"=w233) -> (error out=w251:errorcluster)  [unwired: 1 in, 1 out]
      n198 = property on="Магнитные измерения" class="WFChart (strict)"(error in=w265, "Plot.Visible?"="Plot.Visible Z") -> (error out=w226:errorcluster)  [unwired: 1 in, 1 out]
      n199 = property on="Магнитные измерения" class="WFChart (strict)"(error in=w251, "Plot.Point Style"=w245) -> (error out=w252:errorcluster)  [unwired: 1 in, 1 out]
      n200 = property on="Магнитные измерения" class="WFChart (strict)"(error in=w252, "Active Plot"=u32 1) -> (error out=w257:errorcluster)  [unwired: 1 in, 1 out]
      n201 = property on="Магнитные измерения" class="WFChart (strict)"(error in=w257, "Plot.Line Width"=w233) -> (error out=w249:errorcluster)  [unwired: 1 in, 1 out]
      n202 = property on="Table num index" class="DigNum (strict)"(error in=w226) -> ("Value"=w224:u32)  [unwired: 1 in, 2 out]
      n203 = Equal To 0?(x=w224) -> (x = 0?=w223:bool)
      n204 = case shown="False" w223 {
        tunnel: [u32 0 ("Table num index") u32 2 ("Table num index")] -> w222
        frame False {
        }
        frame True {
        }
      }
      n205 = property on="Магнитные измерения" class="WFChart (strict)"(error in=w249, "Plot.Point Style"=w245) -> (error out=w250:errorcluster)  [unwired: 1 in, 1 out]
      n206 = property on="Удалить измерение" class="Bool (strict)"("Disabled"=w222) -> (error out=w227:errorcluster)  [unwired: 2 in, 1 out]
      n207 = property on="Магнитные измерения" class="WFChart (strict)"(error in=w250, "Active Plot"=u32 2) -> (error out=w254:errorcluster)  [unwired: 1 in, 1 out]
      n208 = property on="Магнитные измерения" class="WFChart (strict)"(error in=w254, "Plot.Line Width"=w233) -> (error out=w248:errorcluster)  [unwired: 1 in, 1 out]
      n209 = property on="Магнитные измерения" class="WFChart (strict)"(error in=w248, "Plot.Point Style"=w245) -> (error out=w232:errorcluster)  [unwired: 1 in, 1 out]
      n210 = Merge Errors(w232, w227) -> (w230:errorcluster)
      n211 = Wait Until Next ms Multiple(millisecond multiple=u32 2) -> ()  [unwired: 1 out]
      n212 = call <vilib>:"Simple Error Handler.vi"("type of dialog (OK msg:1)"=u32 0 ("Table num index"), "error in (no error)"=w230) -> ()  [unwired: 8 out]
    }
  }
